vi "Configure Marker Frequency.vi"(8 "error in (no error)":errorcluster, 9 "Marker Frequency":dbl, 10 "Marker Number":u8=1, 11 "VNA-Keysight PNA in":refnum<class "VNA-Keysight PNA.lvclass">) -> (0 "error out":errorcluster, 3 "VNA-Keysight PNA out":refnum<class "VNA-Keysight PNA.lvclass">)   [LabVIEW 2020, in "VNA-Keysight PNA.lvclass"]
doc: "Configure the marker frequency.\nThe marker is always set on the current active trace."
uses:
  VNA-Keysight PNA.lvclass
  C:/Sandbox/Git_Sandbox/WiSpry Test Framework source code (LV20)/WiSpry Test Framework/Instruments/Instrument.lvclass
  Instrument.lvclass/Instrument.ctl
  Instrument.lvclass
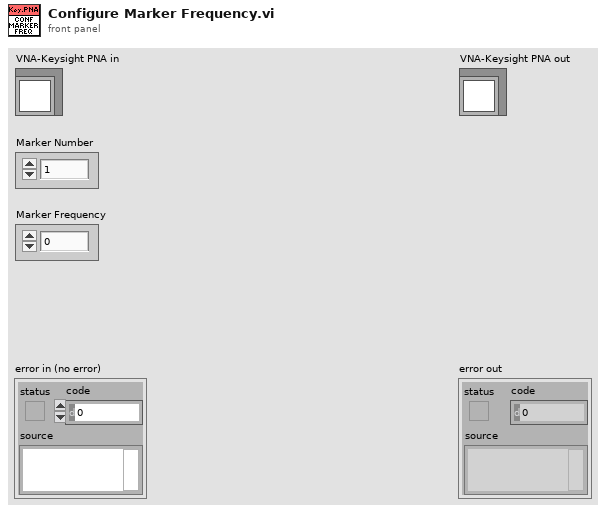
[diagram p1: front panel]
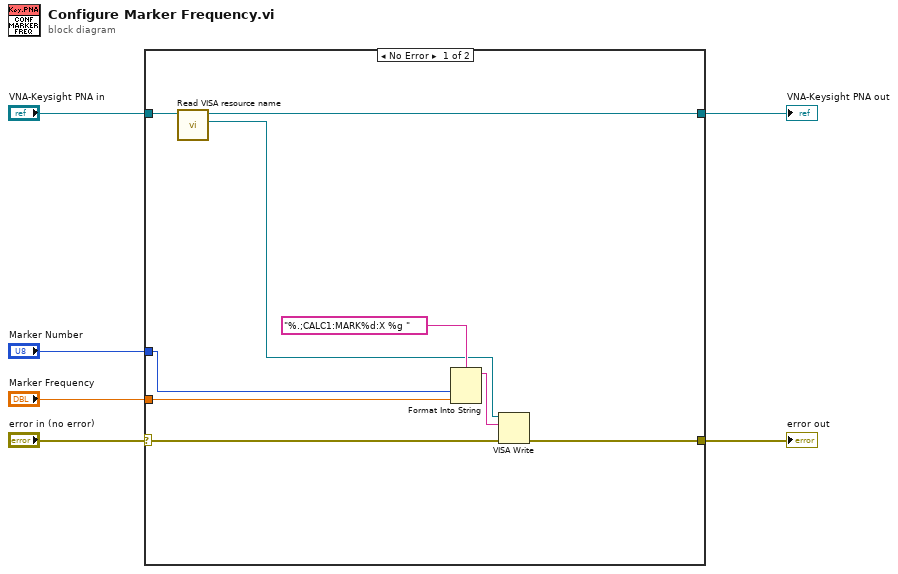
[diagram p0: block diagram]
diagram:
  n1 = case shown="No Error" "error in (no error)" {
    selector: "error in (no error)" -> [w11 w16]
    tunnel: [w14 w17] -> w5
    tunnel: "VNA-Keysight PNA in" -> [w15 w17]
    tunnel: [w10 w16] -> w6
    tunnel: "Marker Frequency" -> [w9 _]
    tunnel: "Marker Number" -> [w8 _]
    frame No Error {
      n2 = call "Read VISA resource name.vi"("Instrument in"=w15) -> ("VISA resource name"=w7:refnum<visa-resource-name>, "Instrument out"=w14:refnum<class "VNA-Keysight PNA.lvclass">)  [unwired: 9 in]
      n3 = Format Into String(format string="%.;CALC1:MARK%d:X %g ", w8, w9) -> (resulting string=w12:string)  [unwired: 2 in, 1 out]
      n4 = VISA Write(VISA resource name=w7, write buffer=w12, error in (no error)=w11) -> (error out=w10:errorcluster)  [unwired: 2 out]
    }
    frame Error {
    }
  }
  "error out" <- w6
  "VNA-Keysight PNA out" <- w5
